vi "Carga Inventario Inicial.vi"(8 "error in (no error)":errorcluster) -> (0 "error out":errorcluster, 3 "Inventario":string[][](array[string]))   [LabVIEW 2020, in "ProductControl.lvlib"]
uses:
  ProductControl.lvlib
  <vilib>/Utility/config.llb/Read Key (String).vi
  <vilib>/Utility/config.llb/NI_LVConfig.lvlib
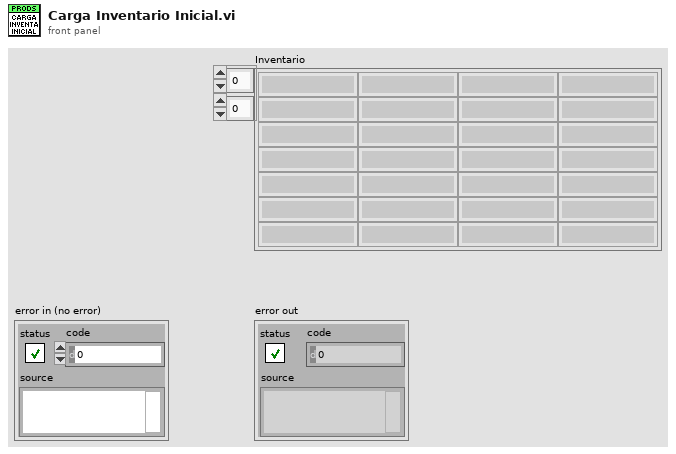
[diagram p1: front panel]
types:
  T1 = typedef "NI_LVConfig.lvlib/Config Data RefNum.ctl" = refnum<k1>
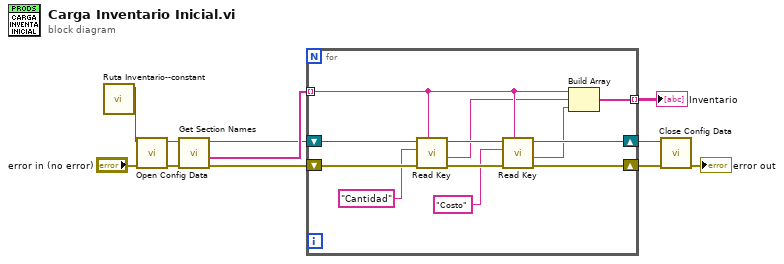
[diagram p0: block diagram]
diagram:
  n1 = call "Ruta Inventario--constant.vi"() -> ("Ruta Inventario"=w6:path)  [unwired: 11 in]
  n2 = call <vilib>:"Open Config Data.vi"("error in (no error)"="error in (no error)", "configuration file path"=w6) -> ("error out"=w11:errorcluster, "refnum"=w5:T1)  [unwired: 7 in, 1 out]
  n3 = call <vilib>:"Get Section Names.vi"("error in (no error)"=w11, "refnum"=w5) -> ("error out"=w10:errorcluster, "section names"=w4:string[], "refnum out"=w3:T1)  [unwired: 7 in]
  n4 = for {
    tunnel: w4 -> [w15] mode=indexing
    shift-right: [w18] -> w2
    shift-left: w3 -> [w19]
    shift-right: [w22] -> w9
    shift-left: w10 -> [w23]
    tunnel: [w12] -> w1 mode=indexing
    n5 = call-poly <vilib>:"Read Key.vi"("section"=w15, "error in (no error)"=w23, "key"="Cantidad", "refnum"=w19) -> ("error out"=w21:errorcluster, "value"=w14:string, "refnum out"=w20:T1)  [unwired: 4 in, 1 out]
    n6 = call-poly <vilib>:"Read Key.vi"("section"=w15, "error in (no error)"=w21, "key"="Costo", "refnum"=w20) -> ("error out"=w22:errorcluster, "value"=w13:string, "refnum out"=w18:T1)  [unwired: 4 in, 1 out]
    n7 = Build Array(w15, w14, w13) -> (w12:string[])
  }
  "Inventario" <- w1
  n8 = call <vilib>:"Close Config Data.vi"("error in (no error)"=w9, "refnum"=w2) -> ("error out"=→"error out":errorcluster)  [unwired: 8 in, 1 out]
